vi "Parse Postfix (RPN) String.vi"() -> ()   [LabVIEW 2020]
doc: "This example VI shows how to use the Scan String for Tokens and Scan From String functions to write a postfix (RPN) expression parser. RPN stands for \"Reverse Polish Notation\"."
panel:
  out "Result":dbl format="%.6f"
  in  "Postfix (RPN) String":string="1 3.1415 2 2 * * +"
  # "Overview: Demonstrates how the Scan String for Tokens function can parse a Postfix (Reverse Polish Notation) string.\nInstructions:\n1. Specify a Postfix (RPN) String. This example recognizes the following operators: *, /, %, +, or -.\n2. Run the VI to display the Result of the RPN calculation."
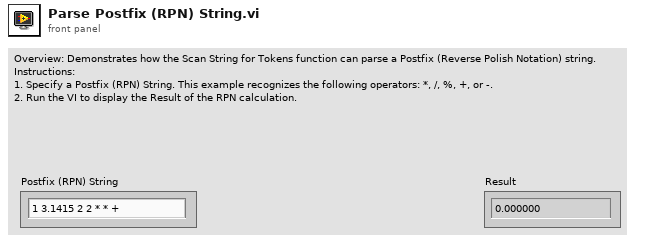
[diagram p1: front panel]
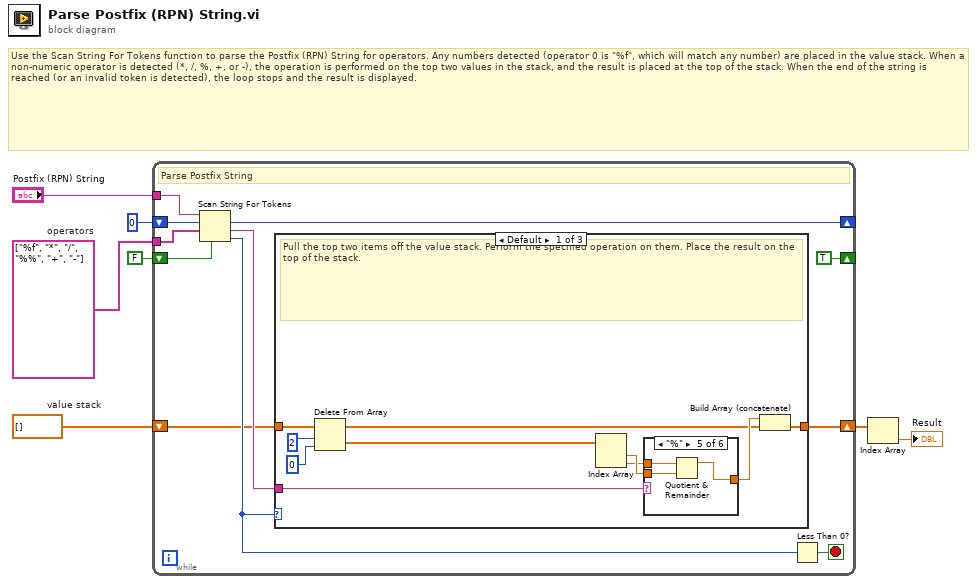
[diagram p0: block diagram]
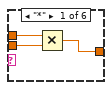
[diagram p2: hidden frame]
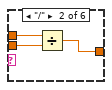
[diagram p3: hidden frame]
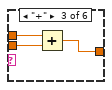
[diagram p4: hidden frame]
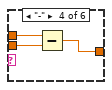
[diagram p5: hidden frame]
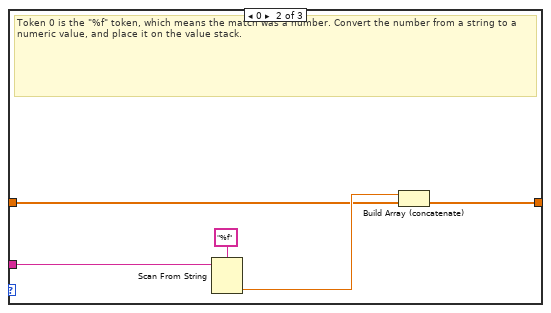
[diagram p7: hidden frame]
diagram:
  w1 = string[] ["%f", "*", "/", "%%", "+", "-"]  # operators
  w4 = dbl[] []  # value stack
  # "Use the Scan String For Tokens function to parse the Postfix (RPN) String for operators. Any numbers detected (operator 0 is \"%f\", which will match any number) are placed in the value stack. When a non-numeric operator is detected (*, /, %, +, or -), the operation is performed on the top two values in the stack, and the result is placed at the top of the stack. When the end of the string is reached (or an invalid token is detected), the loop stops and the result is displayed."
  n1 = while {
    shift-left: w4 -> [w8]
    shift-right: [w11] -> w3
    tunnel: w1 -> [w12]
    tunnel: "Postfix (RPN) String" -> [w14]
    shift-left: FALSE -> [w16]
    shift-right: [TRUE] -> _
    shift-left: 0 ("offset past token") -> [w15]
    shift-right: [w18] -> _
    stop <- w13 stop-if-true
    # "Parse Postfix String"
    n2 = Scan String For Tokens(4:w16, 7:w12, 8:w15, 9:w14) -> (0:w10:i32, 1:w9:string, 2:w18:i32)  [unwired: 2 in, 1 out]
    n3 = case shown="Default" w10 {
      tunnel: w9 -> [w27 w49 _]
      tunnel: [w28 w48 w50] -> w11
      tunnel: w8 -> [w25 w45 w50]
      frame Default {
        # "Pull the top two items off the value stack. Perform the specified operation on them. Place the result on the top of the stack."
        n4 = Delete From Array(array=w25, length=2, index=0) -> (deleted portion=w22:dbl[], array with subset deleted=w23:dbl[])
        n5 = Index Array(array=w22) -> (element #1=w20:dbl, element #2=w19:dbl)  [unwired: 2 in]
        n6 = case shown="\"%\"" w27 {
          tunnel: [w31 w34 w37 w40 w41 w44] -> w26
          tunnel: w20 -> [w30 w33 w36 w39 w43 _]
          tunnel: w19 -> [w29 w32 w35 w38 w42 w44]
          frame "*" {
            n7 = Multiply(x=w29, y=w30) -> (x*y=w31:dbl)
          }
          frame "/" {
            n8 = Divide(x=w32, y=w33) -> (x/y=w34:dbl)
          }
          frame "+" {
            n9 = Add(x=w35, y=w36) -> (x+y=w37:dbl)
          }
          frame "-" {
            n10 = Subtract(x=w38, y=w39) -> (x-y=w40:dbl)
          }
          frame "%" {
            n11 = Quotient & Remainder(x=w42, y=w43) -> (x-y*floor(x/y)=w41:dbl)  [unwired: 1 out]
          }
          frame Default {
          }
        }
        n12 = Build Array (concatenate)(w26, w23) -> (w28:dbl[])
      }
      frame 0 {
        # "Token 0 is the \"%f\" token, which means the match was a number. Convert the number from a string to a numeric value, and place it on the value stack."
        n13 = Scan From String(format string="%f", input string=w49) -> (output 1=w46:dbl)  [unwired: 3 in, 3 out]
        n14 = Build Array (concatenate)(w46, w45) -> (w48:dbl[])
      }
      frame -2, -1 {
        # "No matches. Either an invalid string was detected (-1), or the end of the string was reached (-2), so stop the loop."
      }
    }
    n15 = Less Than 0?(x=w10) -> (x < 0?=w13:bool)
  }
  n16 = Index Array(array=w3) -> (element=→"Result":dbl)  [unwired: 1 in]
